vi "SVPWMalphabetaSGL.vi"(0 "alpha":sgl caption="voltage alpha", 1 "SVPWM_SGL":T1={"max"=0.9999695, "Period"=0, "Deadtime"=1}, 5 "beta":sgl caption="voltage beta", 9 "input valid":bool=TRUE, 12 "enable":bool=TRUE) -> (4 "SwitchPositions":T2, 14 "Sector":u8, 15 "ready for input":bool)   [LabVIEW 2015, in "SVPWM.lvlib"]
uses:
  SVPWM.lvlib
  SwitchPositions.ctl
  SVPWM_SGL.ctl
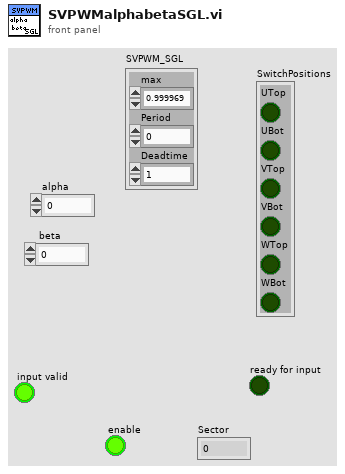
[diagram p1: front panel]
types:
  T1 = typedef "SVPWM.lvlib/SVPWM_SGL.ctl" = cluster{"max":sgl, "Period":u32, "Deadtime":u8}
  T2 = typedef "SVPWM.lvlib/SwitchPositions.ctl" = cluster{"UTop":bool, "UBot":bool, "VTop":bool, "VBot":bool, "WTop":bool, "WBot":bool}
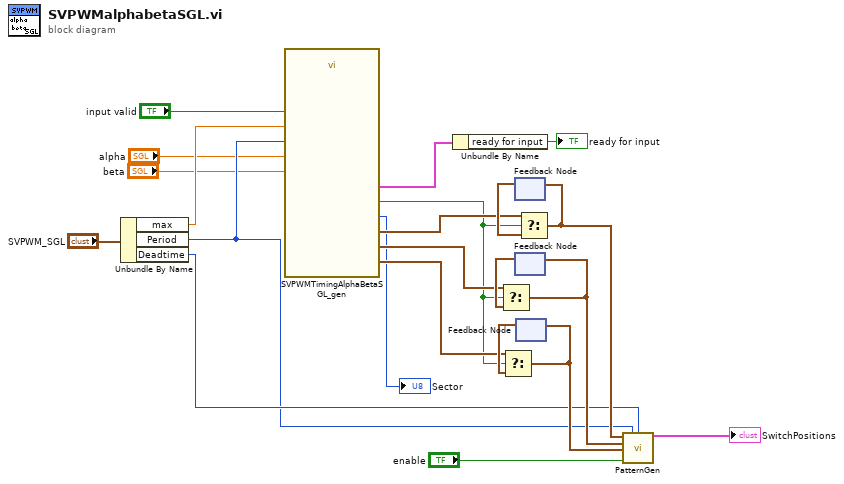
[diagram p0: block diagram]
diagram:
  n1 = Unbundle By Name("SVPWM_SGL") -> ("max"=w7:sgl, "Period"=w3:u32, "Deadtime"=w13:u8)
  n2 = call "SVPWMTimingAlphaBetaSGL_gen.vi"("beta"="beta", "Period"=w3, "max"=w7, "input valid"="input valid", "alpha"="alpha") -> ("Sector"=→"Sector":u8, "W_timing"=w6:cluster{"ON":u32, "OFF":u32}, "V_Timing"=w8:cluster{"ON":u32, "OFF":u32}, "output valid"=w4:bool, "feedback signals"=w9:cluster{"ready for input":bool}, "U_Timing"=w10:cluster{"ON":u32, "OFF":u32})  [unwired: 5 in]
  n3 = Unbundle By Name(w9) -> ("ready for input"=→"ready for input":bool)
  n4 = feedback #1() -> (w22:cluster{"ON":u32, "OFF":u32})  [unwired: 1 in]
  n5 = feedback #2() -> (w21:cluster{"ON":u32, "OFF":u32})  [unwired: 1 in]
  n6 = Select(t=w8, s=w4, f=w21) -> (s? t:f=w18:cluster{"ON":u32, "OFF":u32})
  n7 = feedback-in #2(w18) -> ()
  n8 = feedback #3() -> (w20:cluster{"ON":u32, "OFF":u32})  [unwired: 1 in]
  n9 = Select(t=w6, s=w4, f=w20) -> (s? t:f=w17:cluster{"ON":u32, "OFF":u32})
  n10 = feedback-in #3(w17) -> ()
  n11 = Select(t=w10, s=w4, f=w22) -> (s? t:f=w19:cluster{"ON":u32, "OFF":u32})
  n12 = feedback-in #1(w19) -> ()
  n13 = call "PatternGen.vi"("U_timing"=w19, "Period"=w3, "Deadtime"=w13, "V_timing"=w18, "W_timing"=w17, "enable"="enable") -> ("SwitchPositions"=→"SwitchPositions":T2)  [unwired: 9 in]
